vi "main.vi"() -> ()   [LabVIEW 2023]
panel:
  out "MFD_StatusText":picture
  out "error out":errorcluster
  in  "Connection Type":enum32{"TCP", "SERIAL", "UDP"}(tab)
  in  "tcp":cluster{"address":string, "port":u16}={"address"="127.0.0.1", "port"=5760}
  in  "serial":T1={"baudrate"=115200, "visa in"=""}
  in  "PFD_AirSpeedMinMax":cluster{"Max":i16, "Min":i16, "Show":bool}={"Max"=6, "Min"=0, "Show"=TRUE}
  out "PFD_Top":picture
  out "PFD_HeadingTop":picture
  out "PFD_Heading":picture
  out "PFD_HeadingBack":picture
  out "PFD_AltMid":picture
  out "PFD_AltShort":picture
  out "PFD_Alt":picture
  out "PFD_Airspeed":picture
  out "PFD_Attitude":picture
  in  "Refresh Rate (Hz)":u32=30
  in  "STOP":bool
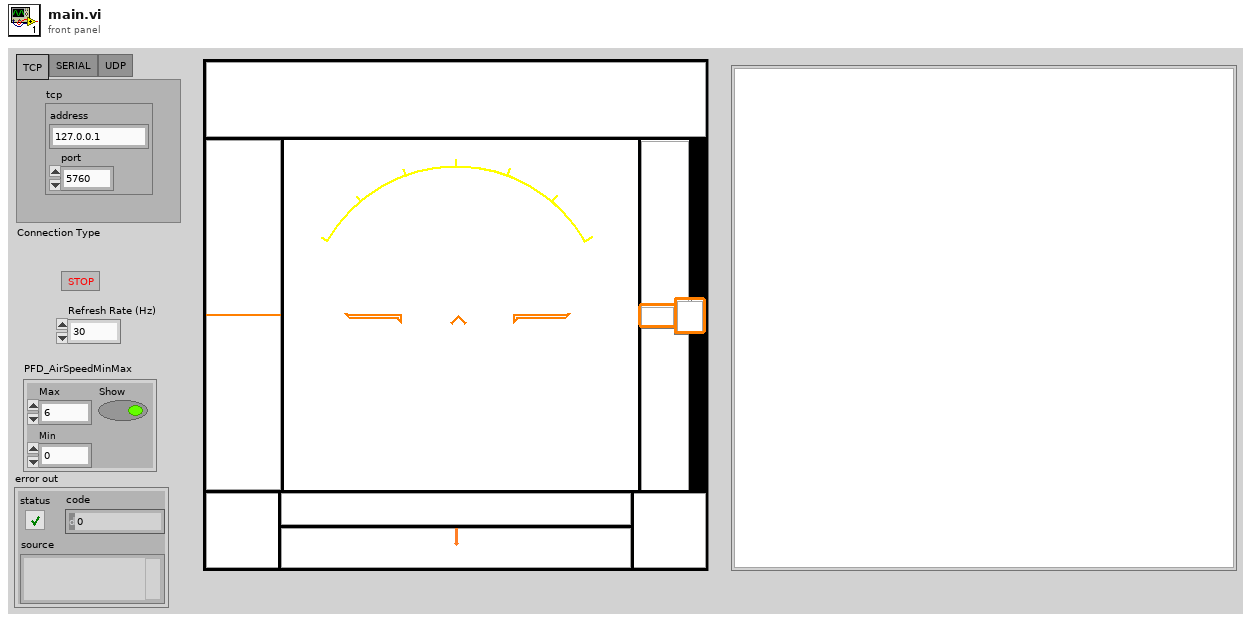
[diagram p1: front panel]
types:
  T1 = cluster{"baudrate":u32, "visa in":refnum<visa-resource-name>}
  T2 = cluster{"HEARTBEAT":cluster{"type":enum8{"MAV_TYPE_GENERIC", "MAV_TYPE_FIXED_WING", "MAV_TYPE_QUADROTOR", "MAV_TYPE_COAXIAL", "MAV_TYPE_HELICOPTER", "MAV_TYPE_ANTENNA_TRACKER", "MAV_TYPE_GCS", "MAV_TYPE_AIRSHIP", "MAV_TYPE_FREE_BALLOON", "MAV_TYPE_ROCKET", "MAV_TYPE_GROUND_ROVER", "MAV_TYPE_SURFACE_BOAT", "MAV_TYPE_SUBMARINE", "MAV_TYPE_HEXAROTOR", "MAV_TYPE_OCTOROTOR", "MAV_TYPE_TRICOPTER", "MAV_TYPE_FLAPPING_WING", "MAV_TYPE_KITE", "MAV_TYPE_ONBOARD_CONTROLLER", "MAV_TYPE_VTOL_TAILSITTER_DUOROTOR", "MAV_TYPE_VTOL_TAILSITTER_QUADROTOR", "MAV_TYPE_VTOL_TILTROTOR", "MAV_TYPE_VTOL_FIXEDROTOR", "MAV_TYPE_VTOL_TAILSITTER", "MAV_TYPE_VTOL_TILTWING", "MAV_TYPE_VTOL_RESERVED5", "MAV_TYPE_GIMBAL", "MAV_TYPE_ADSB", "MAV_TYPE_PARAFOIL", "MAV_TYPE_DODECAROTOR", "MAV_TYPE_CAMERA", "MAV_TYPE_CHARGING_STATION", "MAV_TYPE_FLARM", "MAV_TYPE_SERVO", "MAV_TYPE_ODID", "MAV_TYPE_DECAROTOR", "MAV_TYPE_BATTERY", "MAV_TYPE_PARACHUTE", "MAV_TYPE_LOG", "MAV_TYPE_OSD", "MAV_TYPE_IMU", "MAV_TYPE_GPS", "MAV_TYPE_WINCH", "MAV_TYPE_GENERIC_MULTIROTOR", "MAV_TYPE_ILLUMINATOR"}, "autopilot":enum8{"MAV_AUTOPILOT_GENERIC", "MAV_AUTOPILOT_RESERVED", "MAV_AUTOPILOT_SLUGS", "MAV_AUTOPILOT_ARDUPILOTMEGA", "MAV_AUTOPILOT_OPENPILOT", "MAV_AUTOPILOT_GENERIC_WAYPOINTS_ONLY", "MAV_AUTOPILOT_GENERIC_WAYPOINTS_AND_SIMPLE_NAVIGATION_ONLY", "MAV_AUTOPILOT_GENERIC_MISSION_FULL", "MAV_AUTOPILOT_INVALID", "MAV_AUTOPILOT_PPZ", "MAV_AUTOPILOT_UDB", "MAV_AUTOPILOT_FP", "MAV_AUTOPILOT_PX4", "MAV_AUTOPILOT_SMACCMPILOT", "MAV_AUTOPILOT_AUTOQUAD", "MAV_AUTOPILOT_ARMAZILA", "MAV_AUTOPILOT_AEROB", "MAV_AUTOPILOT_ASLUAV", "MAV_AUTOPILOT_SMARTAP", "MAV_AUTOPILOT_AIRRAILS", "MAV_AUTOPILOT_REFLEX"}, "custom_mode":u32, "system_status":enum16{"MAV_STATE_UNINIT", "MAV_STATE_BOOT", "MAV_STATE_CALIBRATING", "MAV_STATE_STANDBY", "MAV_STATE_ACTIVE", "MAV_STATE_CRITICAL", "MAV_STATE_EMERGENCY", "MAV_STATE_POWEROFF", "MAV_STATE_FLIGHT_TERMINATION"}, "mavlink_version":u8, "base_mode":cluster{"CUSTOM_MODE_ENABLED":bool, "TEST_ENABLED":bool, "AUTO_ENABLED":bool, "GUIDED_ENABLED":bool, "STABILIZE_ENABLED":bool, "HIL_ENABLED":bool, "MANUAL_INPUT_ENABLED":bool, "SAFETY_ARMED":bool}, "HEARTBEAT_TIMER":u32, "copter_flight_mode":enum32{"Stabilize", "Acro", "AltHold", "Auto", "Guided", "Loiter", "RTL", "Circle", "--Deprecated-8", "Land", "--Deprecated-10", "Drift", "--Deprecated-12", "Sport", "Flip", "AutoTune", "PosHold", "Brake", "Throw", "Avoid_ADSB", "Guided_NoGPS", "Smart_RTL", "FlowHold", "Follow", "ZigZag", "SystemID", "Heli_Autorotate", "Auto RTL"}}, "Batt Stats":cluster{"Active":bool, "State":bool}, "Sat Stats":cluster{"Active":bool, "State":bool}, "Radio Stats":cluster{"Active":bool, "State":bool}, "Sensor Stats":cluster{"Active":bool, "State":bool}}
  T3 = cluster{"type":enum8{"MAV_TYPE_GENERIC", "MAV_TYPE_FIXED_WING", "MAV_TYPE_QUADROTOR", "MAV_TYPE_COAXIAL", "MAV_TYPE_HELICOPTER", "MAV_TYPE_ANTENNA_TRACKER", "MAV_TYPE_GCS", "MAV_TYPE_AIRSHIP", "MAV_TYPE_FREE_BALLOON", "MAV_TYPE_ROCKET", "MAV_TYPE_GROUND_ROVER", "MAV_TYPE_SURFACE_BOAT", "MAV_TYPE_SUBMARINE", "MAV_TYPE_HEXAROTOR", "MAV_TYPE_OCTOROTOR", "MAV_TYPE_TRICOPTER", "MAV_TYPE_FLAPPING_WING", "MAV_TYPE_KITE", "MAV_TYPE_ONBOARD_CONTROLLER", "MAV_TYPE_VTOL_TAILSITTER_DUOROTOR", "MAV_TYPE_VTOL_TAILSITTER_QUADROTOR", "MAV_TYPE_VTOL_TILTROTOR", "MAV_TYPE_VTOL_FIXEDROTOR", "MAV_TYPE_VTOL_TAILSITTER", "MAV_TYPE_VTOL_TILTWING", "MAV_TYPE_VTOL_RESERVED5", "MAV_TYPE_GIMBAL", "MAV_TYPE_ADSB", "MAV_TYPE_PARAFOIL", "MAV_TYPE_DODECAROTOR", "MAV_TYPE_CAMERA", "MAV_TYPE_CHARGING_STATION", "MAV_TYPE_FLARM", "MAV_TYPE_SERVO", "MAV_TYPE_ODID", "MAV_TYPE_DECAROTOR", "MAV_TYPE_BATTERY", "MAV_TYPE_PARACHUTE", "MAV_TYPE_LOG", "MAV_TYPE_OSD", "MAV_TYPE_IMU", "MAV_TYPE_GPS", "MAV_TYPE_WINCH", "MAV_TYPE_GENERIC_MULTIROTOR", "MAV_TYPE_ILLUMINATOR"}, "autopilot":enum8{"MAV_AUTOPILOT_GENERIC", "MAV_AUTOPILOT_RESERVED", "MAV_AUTOPILOT_SLUGS", "MAV_AUTOPILOT_ARDUPILOTMEGA", "MAV_AUTOPILOT_OPENPILOT", "MAV_AUTOPILOT_GENERIC_WAYPOINTS_ONLY", "MAV_AUTOPILOT_GENERIC_WAYPOINTS_AND_SIMPLE_NAVIGATION_ONLY", "MAV_AUTOPILOT_GENERIC_MISSION_FULL", "MAV_AUTOPILOT_INVALID", "MAV_AUTOPILOT_PPZ", "MAV_AUTOPILOT_UDB", "MAV_AUTOPILOT_FP", "MAV_AUTOPILOT_PX4", "MAV_AUTOPILOT_SMACCMPILOT", "MAV_AUTOPILOT_AUTOQUAD", "MAV_AUTOPILOT_ARMAZILA", "MAV_AUTOPILOT_AEROB", "MAV_AUTOPILOT_ASLUAV", "MAV_AUTOPILOT_SMARTAP", "MAV_AUTOPILOT_AIRRAILS", "MAV_AUTOPILOT_REFLEX"}, "custom_mode":u32, "system_status":enum16{"MAV_STATE_UNINIT", "MAV_STATE_BOOT", "MAV_STATE_CALIBRATING", "MAV_STATE_STANDBY", "MAV_STATE_ACTIVE", "MAV_STATE_CRITICAL", "MAV_STATE_EMERGENCY", "MAV_STATE_POWEROFF", "MAV_STATE_FLIGHT_TERMINATION"}, "mavlink_version":u8, "base_mode":cluster{"CUSTOM_MODE_ENABLED":bool, "TEST_ENABLED":bool, "AUTO_ENABLED":bool, "GUIDED_ENABLED":bool, "STABILIZE_ENABLED":bool, "HIL_ENABLED":bool, "MANUAL_INPUT_ENABLED":bool, "SAFETY_ARMED":bool}, "HEARTBEAT_TIMER":u32, "copter_flight_mode":enum32{"Stabilize", "Acro", "AltHold", "Auto", "Guided", "Loiter", "RTL", "Circle", "--Deprecated-8", "Land", "--Deprecated-10", "Drift", "--Deprecated-12", "Sport", "Flip", "AutoTune", "PosHold", "Brake", "Throw", "Avoid_ADSB", "Guided_NoGPS", "Smart_RTL", "FlowHold", "Follow", "ZigZag", "SystemID", "Heli_Autorotate", "Auto RTL"}}
  T4 = cluster{"time_boot_ms":u32, "roll":sgl, "pitch":sgl, "yaw":sgl, "rollspeed":sgl, "pitchspeed":sgl, "yawspeed":sgl}
  T5 = cluster{"airspeed (m/s)":sgl, "groundspeed (m/s)":sgl, "heading (deg) ":i16, "throttle (%) ":u16, "alt (m)":sgl, "climb (m/s)":sgl}
  T6 = cluster{"time_boot_ms":u32, "lat":i32, "lon":i32, "alt (mm) [MSL]":i32, "relative_alt (above gnd)":i32, "vx":i16, "vy":i16, "vz":i16, "hdg":u16}
  T7 = cluster{"severity":enum8{"MAV_SEVERITY_EMERGENCY", "MAV_SEVERITY_ALERT", "MAV_SEVERITY_CRITICAL", "MAV_SEVERITY_ERROR", "MAV_SEVERITY_WARNING", "MAV_SEVERITY_NOTICE", "MAV_SEVERITY_INFO", "MAV_SEVERITY_DEBUG"}, "id":u16, "chunk_seq":u8, "text":string}[]
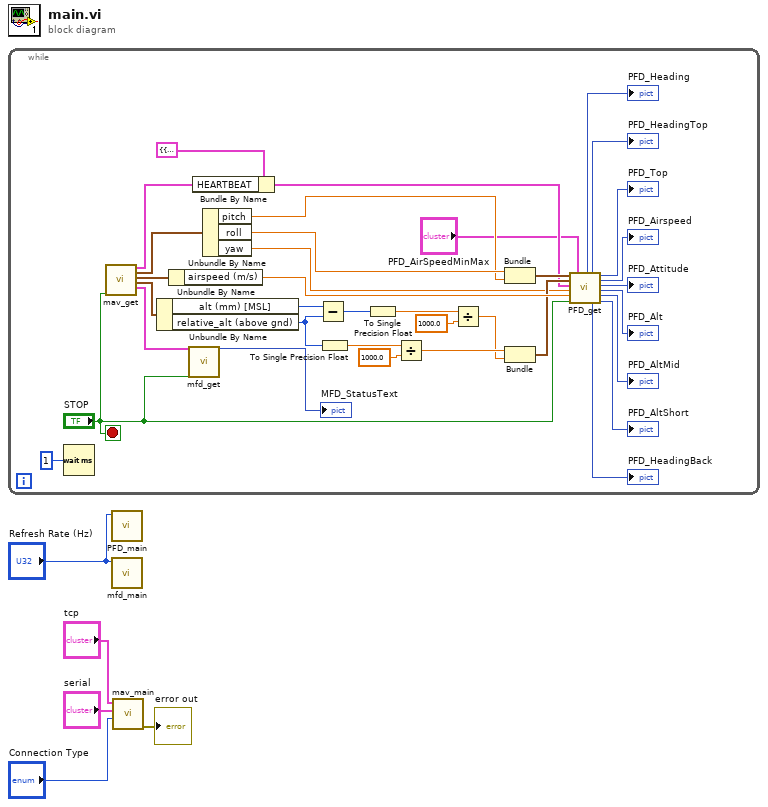
[diagram p0: block diagram]
diagram:
  n1 = while {
    stop <- "STOP" stop-if-true
    n2 = Wait (ms)(milliseconds to wait=u32 1) -> ()  [unwired: 1 out]
    n3 = call "mav_get.vi"("stop"="STOP") -> ("HEARTBEAT #0"=w27:T3, "ATTITUDE #30"=w31:T4, "VFR_HUD #74"=w19:T5, "GLOBAL_POSITION_INT #33"=w18:T6, "STATUSTEXT"=w7:T7)  [unwired: 14 in]
    n4 = Unbundle By Name(w18) -> ("alt (mm) [MSL]"=w17:i32, "relative_alt (above gnd)"=w16:i32)
    n5 = Unbundle By Name(w19) -> ("airspeed (m/s)"=w29:sgl)
    n6 = call "mfd_get.vi"("STATUSTEXT"=w7, "MFD_Stop"="STOP") -> ("MFD_StatusText"=→"MFD_StatusText":picture)  [unwired: 25 in]
    n7 = Bundle By Name(cluster=T2 {"HEARTBEAT"={"type"=enum."MAV_TYPE_FIXED_WING", "autopilot"=enum."MAV_AUTOPILOT_AEROB", "custom_mode"=0, "system_status"=enum."MAV_STATE_CRITICAL", "mavlink_version"=0, "base_mode"={"CUSTOM_MODE_ENABLED"=FALSE, "TEST_ENABLED"=FALSE, "AUTO_ENABLED"=FALSE, "GUIDED_ENABLED"=FALSE, "STABILIZE_ENABLED"=FALSE, "HIL_ENABLED"=FALSE, "MANUAL_INPUT_ENABLED"=FALSE, "SAFETY_ARMED"=FALSE}, "HEARTBEAT_TIMER"=0, "copter_flight_mode"=enum."Stabilize"}, "Batt Stats"={"Active"=TRUE, "State"=FALSE}, "Sat Stats"={"Active"=TRUE, "State"=FALSE}, "Radio Stats"={"Active"=TRUE, "State"=FALSE}, "Sensor Stats"={"Active"=TRUE, "State"=FALSE}} ("PFD_TopControl"), "HEARTBEAT"=w27) -> (w23:T2)
    n8 = Unbundle By Name(w31) -> ("pitch"=w25:sgl, "roll"=w26:sgl, "yaw"=w22:sgl)
    n9 = Subtract(x=w17, y=w16) -> (x-y=w12:i32)
    n10 = To Single Precision Float(number=w16) -> (single precision float=w15:sgl)
    n11 = To Single Precision Float(number=w12) -> (single precision float=w10:sgl)
    n12 = Divide(x=w15, y=sgl 1000.0) -> (x/y=w13:sgl)
    n13 = Divide(x=w10, y=sgl 1000.0) -> (x/y=w9:sgl)
    n14 = Bundle("roll"=w26, "pitch"=w25) -> (w30:cluster{"roll":sgl, "pitch":sgl})  [unwired: 1 in]
    n15 = Bundle(w13, w9) -> (w28:cluster{sgl, sgl})  [unwired: 1 in]
    n16 = call "PFD_get.vi"("PFD_AttitudeControl"=w30, "PFD_AltitudeControl"=w28, "PFD_TopControl"=w23, "PFD_HeadingControl"=w22, "PFD_AirSpeedControl"=w29, "PFD_STOP"="STOP", "PFD_AirSpeedMinMax"="PFD_AirSpeedMinMax") -> ("PFD_Heading"=→"PFD_Heading":picture, "PFD_HeadingTop"=→"PFD_HeadingTop":picture, "PFD_HeadingBack"=→"PFD_HeadingBack":picture, "PFD_Top"=→"PFD_Top":picture, "PFD_Airspeed"=→"PFD_Airspeed":picture, "PFD_Attitude"=→"PFD_Attitude":picture, "PFD_Alt"=→"PFD_Alt":picture, "PFD_AltMid"=→"PFD_AltMid":picture, "PFD_AltShort"=→"PFD_AltShort":picture)  [unwired: 4 in]
  }
  n17 = call "PFD_main.vi"("Refresh Rate (Hz)"="Refresh Rate (Hz)") -> ()  [unwired: 11 in]
  n18 = call "mfd_main.vi"("Refresh Rate (Hz)"="Refresh Rate (Hz)") -> ()  [unwired: 11 in]
  n19 = call "mav_main.vi"("Connection Type"="Connection Type", "serial"="serial", "tcp"="tcp") -> ("error out"=→"error out":errorcluster)  [unwired: 8 in]
